vi "sData Write.vi"(6 "Slow Timestamp":u64, 8 "error in":errorcluster, 9 "Slow Data":dbl, 10 "Slow ID number":i32, 11 "File in":refnum<file>) -> (0 "error out":errorcluster, 3 "File out":refnum<file>)   [LabVIEW 2012]
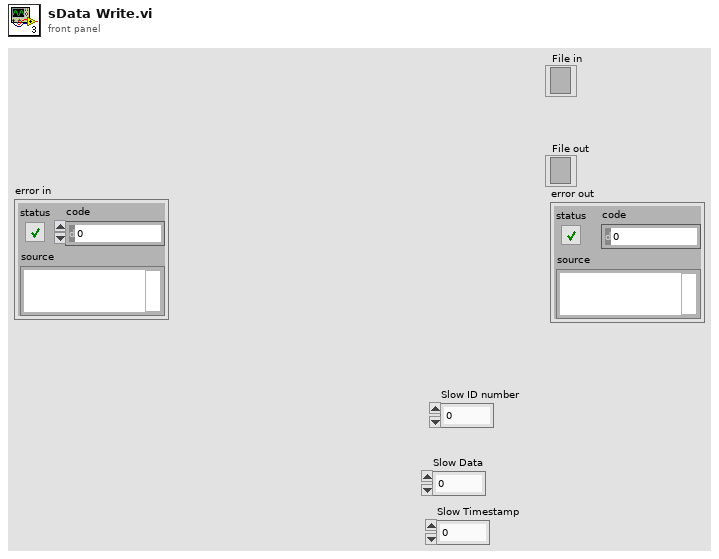
[diagram p1: front panel]
types:
  T1 = enum16{"big-endian, network order", "native, host order", "little-endian"}
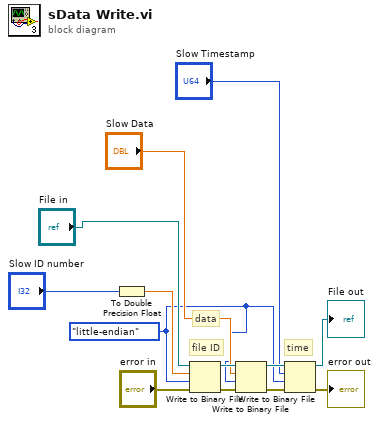
[diagram p0: block diagram]
diagram:
  w1 = T1."little-endian" ("byte order (0:big-endian, network order)")
  # "time"
  # "data"
  # "file ID"
  n1 = To Double Precision Float(number="Slow ID number") -> (double precision float=w4:dbl)
  n2 = Write to Binary File(file (use dialog)="File in", data=w4, error in="error in", 9:w1) -> (refnum out=w12:refnum<file>, error out=w13:errorcluster)  [unwired: 2 in, 1 out]
  n3 = Write to Binary File(file (use dialog)=w12, data="Slow Data", error in=w13, 9:w1) -> (refnum out=w11:refnum<file>, error out=w10:errorcluster)  [unwired: 2 in, 1 out]
  n4 = Write to Binary File(file (use dialog)=w11, data="Slow Timestamp", error in=w10, 9:w1) -> (refnum out=→"File out":refnum<file>, error out=→"error out":errorcluster)  [unwired: 2 in, 1 out]
